vi "getServerRepoId.vi"(8 "error in (no error)":errorcluster, 11 "hgHandler in":refnum<class "hgHandler.lvclass">) -> (0 "error out":errorcluster, 1 "Log":string, 3 "hgHandler out":refnum<class "hgHandler.lvclass">, 4 "ID":string)   [LabVIEW 2013, in "hgHandler.lvclass"]
uses:
  hgHandler.lvclass
  <vilib>/httpClient/LabVIEWHTTPClient.lvlib
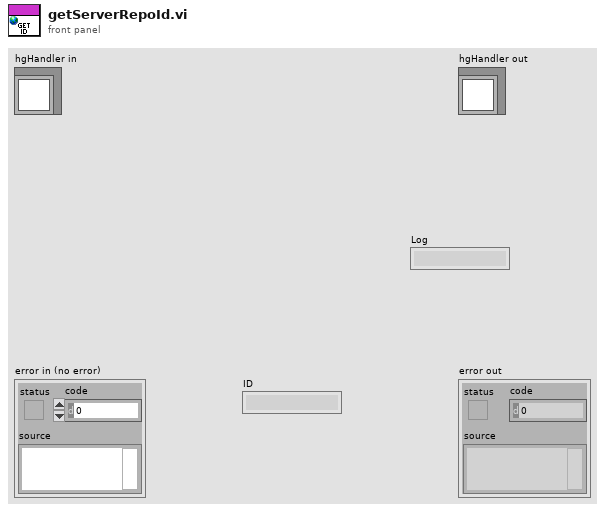
[diagram p1: front panel]
types:
  T1 = typedef "LabVIEWHTTPClient.lvlib/ClientHandle.ctl" = refnum<k1>
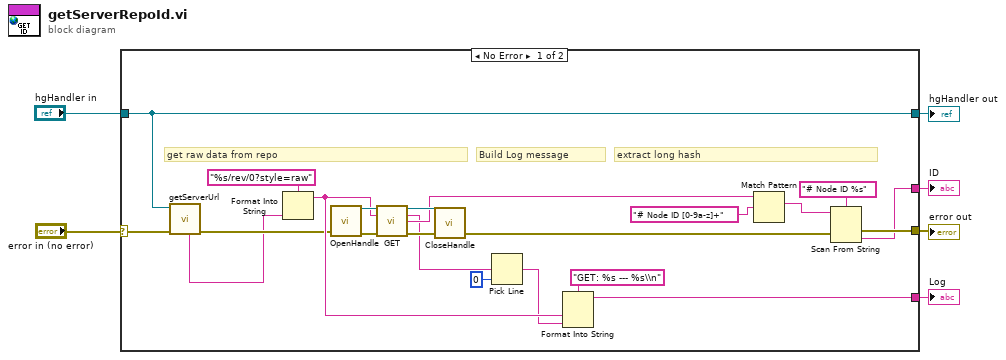
[diagram p0: block diagram]
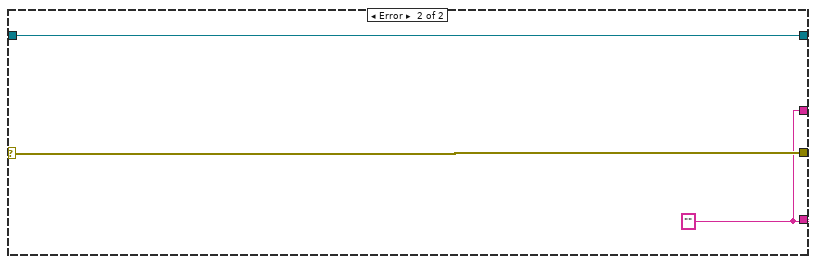
[diagram p2: hidden frame]
diagram:
  n1 = case shown="No Error" "error in (no error)" {
    selector: "error in (no error)" -> [w11 w30]
    tunnel: "hgHandler in" -> [w13 w31]
    tunnel: [w13 w31] -> w4
    tunnel: [w10 w30] -> w3
    tunnel: [w9 w29] -> w2
    tunnel: [w8 w29] -> w1
    frame No Error {
      # "Build Log message"
      # "extract long hash"
      # "get raw data from repo"
      n2 = call-dynamic "getServerUrl.vi"("error in (no error)"=w11, "repoHandler in"=w13) -> ("error out"=w12:errorcluster, "Server url"=w7:string)  [unwired: 7 in, 1 out]
      n3 = Format Into String(format string="%s/rev/0?style=raw", w7) -> (resulting string=w17:string)  [unwired: 2 in, 1 out]
      n4 = call <vilib>:"OpenHandle.vi"("error in (no error)"=w12) -> ("client handle out"=w25:T1, "error out"=w27:errorcluster)  [unwired: 13 in]
      n5 = call <vilib>:"GET.vi"("client handle"=w25, "url"=w17, "error in (no error)"=w27) -> ("client handle out"=w24:T1, "headers"=w15:string, "body"=w23:string, "error out"=w26:errorcluster)  [unwired: 9 in]
      n6 = call <vilib>:"CloseHandle.vi"("client handle"=w24, "error in (no error)"=w26) -> ("error out"=w19:errorcluster)  [unwired: 13 in]
      n7 = Pick Line(multi-line string=w15, line index=0) -> (output string=w14:string)  [unwired: 1 in]
      n8 = Format Into String(format string="GET: %s --- %s\\n", w17, w14) -> (resulting string=w9:string)  [unwired: 2 in, 1 out]
      n9 = Match Pattern(string=w23, regular expression="# Node ID [0-9a-z]+") -> (match substring=w21:string)  [unwired: 1 in, 3 out]
      n10 = Scan From String(format string="# Node ID %s" ("search string/char (-)"), input string=w21, error in=w19) -> (error out=w10:errorcluster, output 1=w8:string)  [unwired: 2 in, 2 out]
    }
    frame Error {
      w29 = ""
    }
  }
  "error out" <- w3
  "hgHandler out" <- w4
  "Log" <- w2
  "ID" <- w1
